vi "Create Logging Config File.vi"() -> ()   [LabVIEW 2014]
uses:
  S7 TCP API Library/S7 Read Write Cluster.ctl
  S7 TCP API Library/S7 TCP.lvlib
  S7 TCP API Library/Data Type.ctl
panel:
  in  "IP Address":string="172.16.102.180"
  in  "S7 Read Write Array":T3(array[cluster])=[{"Description"="", "S7 Read Cluster"={"Read / Write"=4, "Address Areas"=132, "Data Block #"=0, "Start Address (bytes)"=0, "Data Type"=enum."Bit", "Bit Number / Byte Length"=0, "Write Data"=0.0}}] {"S7 Read Cluster"."Address Areas" items=["I/O (P)"=128, "Input (I)"=129, "Output (Q)"=130, "Bit Memory (M)"=131, "Data (DB)"=132, "Instance Data (DI)"=133, "Local Data (L)"=134, "Predecessor Local Data (VL)"=135]; "S7 Read Cluster"."Read / Write" items=["Read"=4, "Write"=5]}
  # "Instructions: Configure channels desired to be logged\nin the S7 Read Write Array. Run the VI and it will \ncreate a csv file with the array data. The VI will prompt \nwhere to save the file."
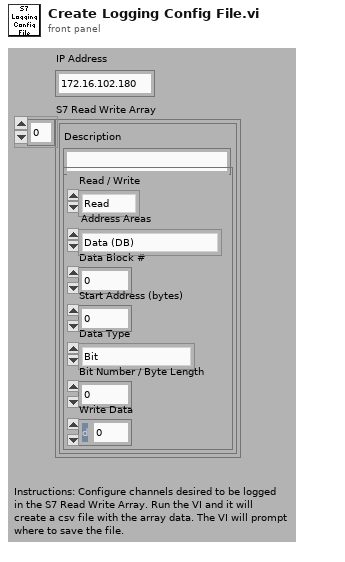
[diagram p1: front panel]
types:
  T1 = typedef "S7 TCP.lvlib/S7 Read Write Cluster.ctl" = cluster{"Read / Write":u8, "Address Areas":u8, "Data Block #":u16, "Start Address (bytes)":u32, "Data Type":T2, "Bit Number / Byte Length":u8, "Write Data":dbl}
  T2 = typedef "S7 TCP.lvlib/Data Type.ctl" = enum16{"Bit", "Byte (U8)", "Signed Byte (I8)", "Word (U16)", "Signed Word (I16)", "Long (U32)", "Signed Long (I32)", "Real (SGL)", "Defined Byte Length"}
  T3 = cluster{"Description":string, "S7 Read Cluster":T1}[]
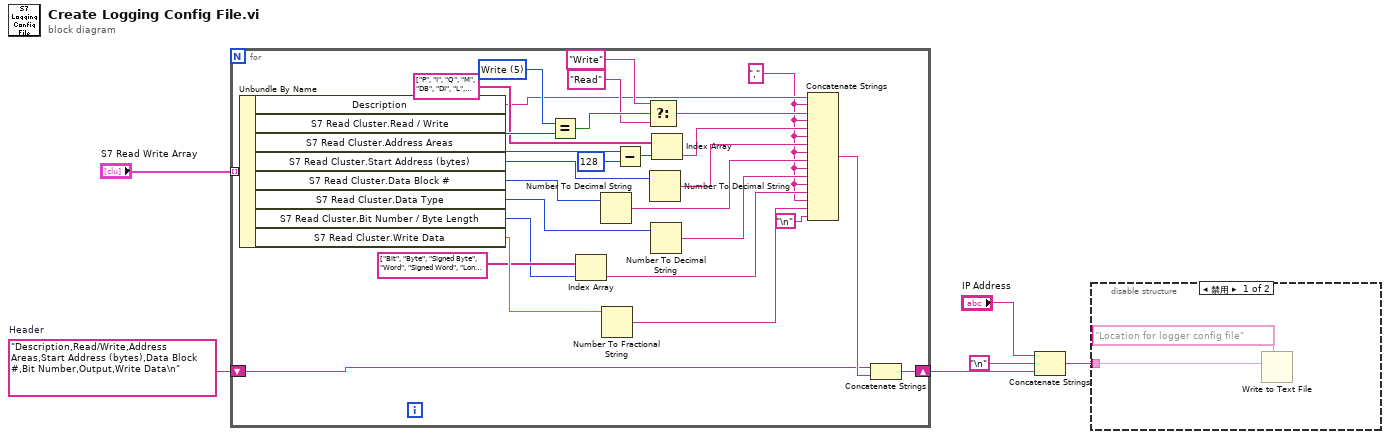
[diagram p0: block diagram]
diagram:
  w5 = "Description,Read/Write,Address Areas,Start Address (bytes),Data Block #,Bit Number,Output,Write Data\n"  # Header
  n1 = for {
    tunnel: "S7 Read Write Array" -> [w35] mode=indexing
    shift-right: [w17] -> w4
    shift-left: w5 -> [w15]
    w7 = "," ("string")
    w34 = u8 5 items=["Read"=4, "Write"=5] ("Read / Write")
    n2 = Unbundle By Name(w35) -> ("Description"=w8:string, "S7 Read Cluster.Read / Write"=w33:u8, "S7 Read Cluster.Address Areas"=w11:u8, "S7 Read Cluster.Start Address (bytes)"=w28:u32, "S7 Read Cluster.Data Block #"=w26:u16, "S7 Read Cluster.Data Type"=w24:T2, "S7 Read Cluster.Bit Number / Byte Length"=w19:u8, "S7 Read Cluster.Write Data"=w22:dbl)
    n3 = Equal?(x=w34, y=w33) -> (x = y?=w32:bool)
    n4 = Index Array(array=string[] ["Bit", "Byte", "Signed Byte", "Word", "Signed Word", "Long", "Signed Long", "Real"] ("Strings []"), index=w19) -> (element=w18:string)
    n5 = Number To Decimal String(number=w26) -> (decimal integer string=w25:string)  [unwired: 1 out]
    n6 = Number To Fractional String(number=w22) -> (F-format string=w21:string)  [unwired: 3 out]
    n7 = Subtract(x=w11, y=u8 128) -> (x-y=w12:u8)
    n8 = Select(t="Write", s=w32, f="Read") -> (s? t:f=w29:string)
    n9 = Number To Decimal String(number=w28) -> (decimal integer string=w27:string)  [unwired: 1 out]
    n10 = Number To Decimal String(number=w24) -> (decimal integer string=w23:string)  [unwired: 1 out]
    n11 = Index Array(array=string[] ["P", "I", "Q", "M", "DB", "DI", "L", "VL"] ("Strings []"), index=w12) -> (element=w14:string)
    n12 = Concatenate Strings(w8, w7, w29, w7, w14, w7, w27, w7, w25, w7, w23, w7, w18, w7, w21, "\n") -> (w16:string)
    n13 = Concatenate Strings(w15, w16) -> (w17:string)
  }
  n14 = Concatenate Strings("IP Address", "\n", w4) -> (w3:string)
  n15 = disable-structure shown="禁用" {
    disable-tunnel: w3 -> [w36 _]
    frame Disabled {
      n16 = Write to Text File(prompt (Choose or enter file path)="Location for logger config file", text=w36) -> ()  [unwired: 1 in, 4 out]
    }
    frame Enabled {
    }
  }
